vi "POST IoT Config Details.vi"(0 "GTron in":path, 3 "error in":errorcluster) -> (6 "IsEmpty":bool, 9 "error out":errorcluster)   [LabVIEW 2019, in "DataLogger.lvclass"]
doc: "POST IoT Configuration Details"
uses:
  DataLogger.lvclass
  <vilib>/drjdpowell/SQLite Library/SQL Connection/Execute SQL (Single Integer).vi
  <vilib>/httpClient/LabVIEWHTTPClient.lvlib
  <vilib>/drjdpowell/SQLite Library/SQL Statement/SQL Statement.lvclass
  <vilib>/drjdpowell/SQLite Library/SQL Connection/Execute SQL (No results).vi
  <vilib>/httpClient/POSTBuffer.vi
  <vilib>/drjdpowell/SQLite Library/SQL Connection/Open (path).vi
  <vilib>/drjdpowell/SQLite Library/SQL Connection/Connection.lvclass
panel:
  in  "IoT_Config Keys in":string[](array[string])=["ClientId", "ClientName", "Location", "NoOfShifts", "RunningShift", "ShiftTiming", "InspectionMcId", "IoTEnable", "SMSAlertEnable", "EmailAlertEnable", "PopUpEnable"]
  in  "Sever Info Cluster fot IoT Config":T1={"JSON Buffer"="authtoken=47244d7c61d7e6141acdddeabbf622d1&scope=creatorapi&zc_ownername=zentron3&XMLString=", "Server information start tag"="<ZohoCreator> <applicationlist> <application name='iiot-gtron'><formlist>  <form name='Iot_Config'>", "Record start/end"="add", "Key name"="field name", "Value name"="value", "Server information end tag"="\"</form></formlist></application></applicationlist></ZohoCreator>"}
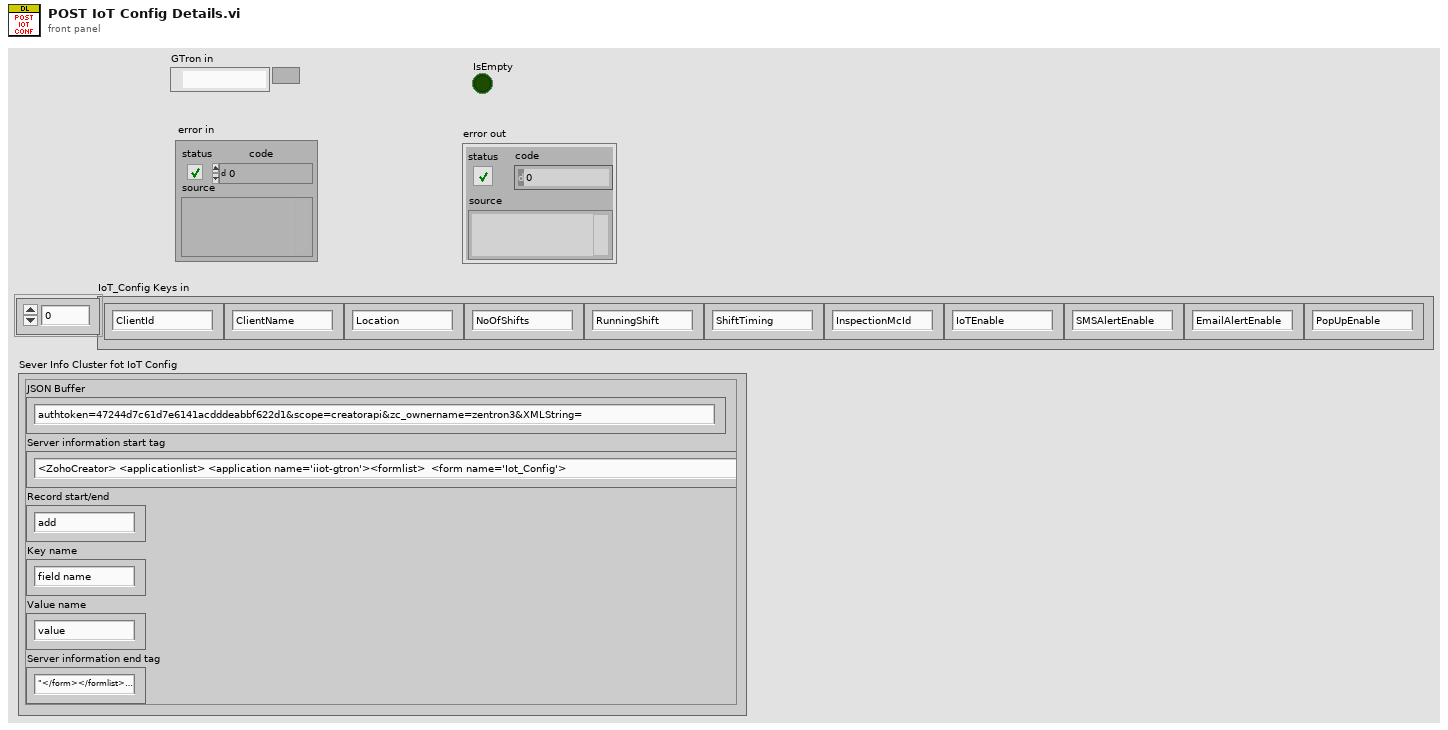
[diagram p1: front panel]
types:
  T1 = cluster{"JSON Buffer":string, "Server information start tag":string, "Record start/end":string, "Key name":string, "Value name":string, "Server information end tag":string}
  T2 = typedef "LabVIEWHTTPClient.lvlib/ClientHandle.ctl" = refnum<k1>
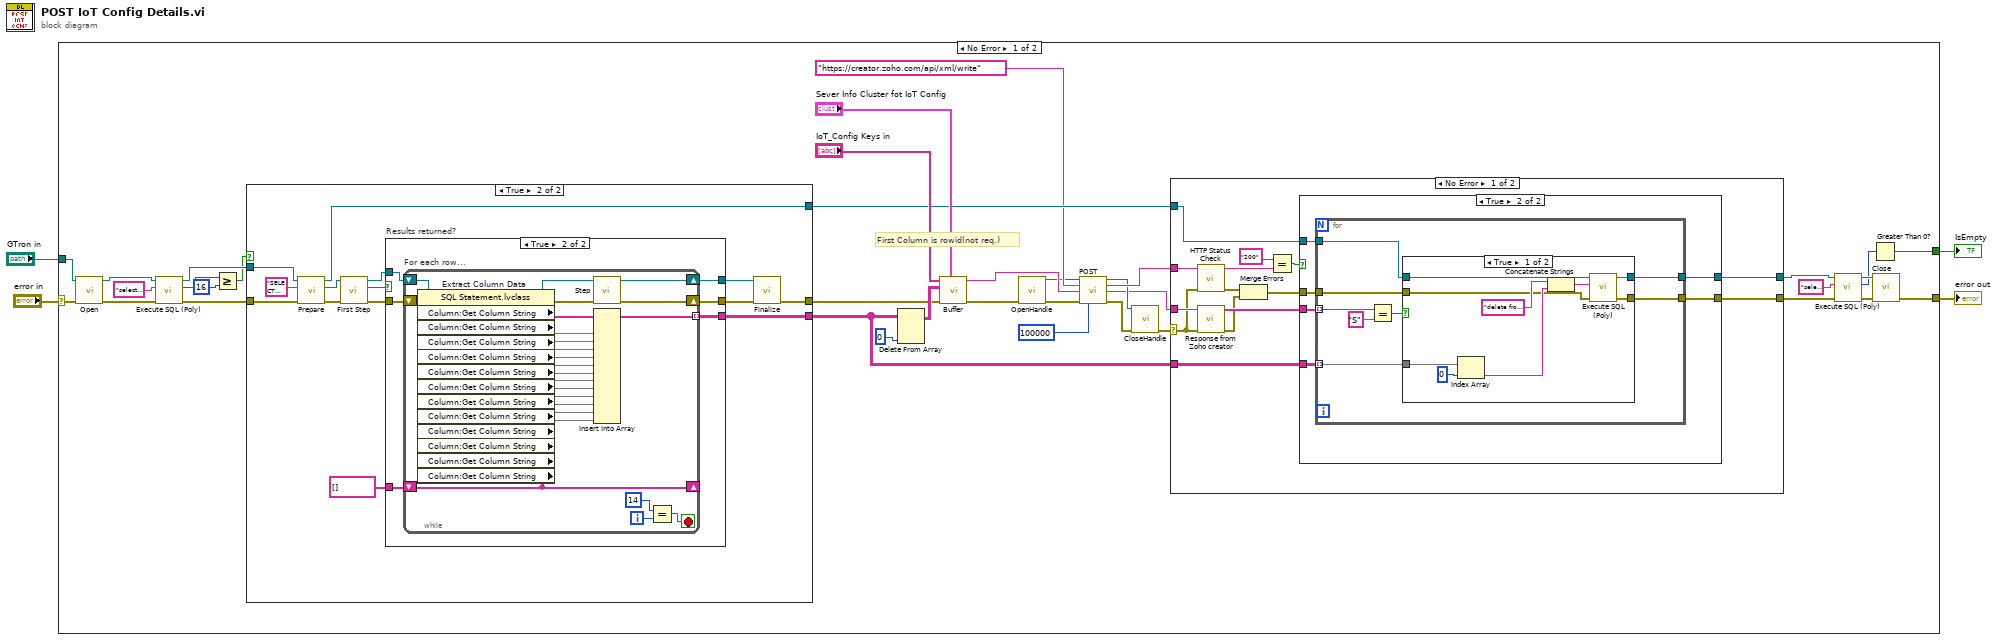
[diagram p0: block diagram]
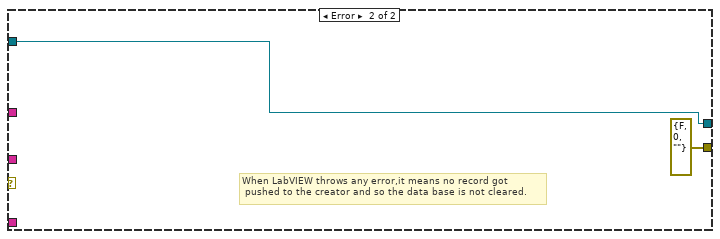
[diagram p4: hidden frame]
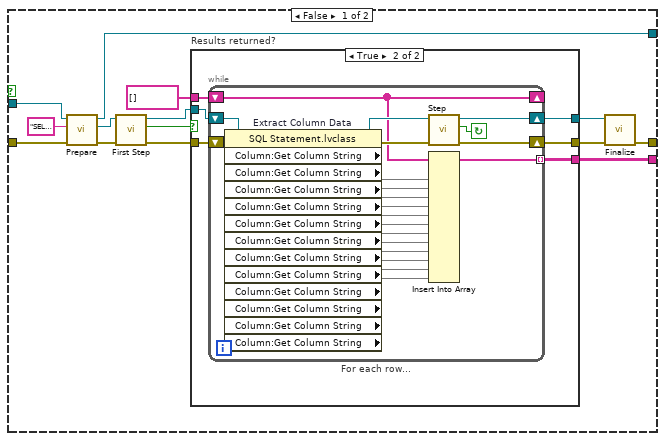
[diagram p5: hidden frame]
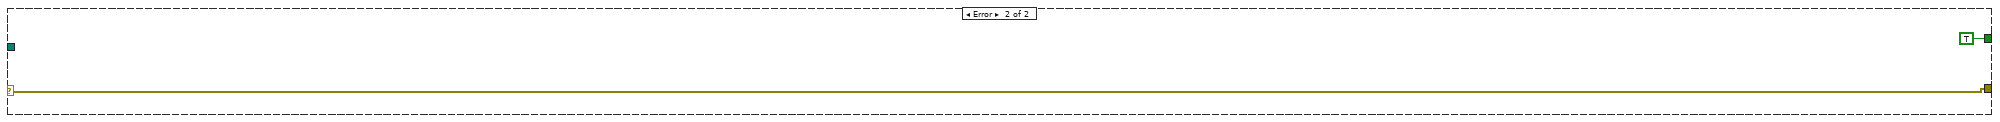
[diagram p8: hidden frame]
diagram:
  n1 = case shown="No Error" "error in" {
    selector: "error in" -> [w5 w172]
    tunnel: "GTron in" -> [w40 _]
    tunnel: [w39 w172] -> w3
    tunnel: [w6 TRUE] -> w2
    frame No Error {
      # "First Column is rowid(not req.)"
      n2 = call-poly <vilib>:"Open.vi"("error in (no error)"=w5, "db file"=w40) -> ("error out"=w37:errorcluster, "SQLite Connection"=w38:refnum<class "Connection.lvclass">)  [unwired: 8 in]
      n3 = call-poly <vilib>:"Execute SQL (Poly).vi"("error in (no error)"=w37, "SQL"="select count(*) from IoTConfigDetails ", "SQLite Connection in"=w38) -> ("error out"=w13:errorcluster, "Result"=w18:i64, "SQLite Connection"=w32:refnum<class "Connection.lvclass">)  [unwired: 6 in]
      n4 = Greater Or Equal?(x=w18, y=i64 16) -> (x >= y?=w20:bool)
      n5 = case shown="True" w20 {
        tunnel: [w89 w132] -> w34
        tunnel: w32 -> [w88 w131]
        tunnel: [w87 w130] -> w33
        tunnel: w13 -> [w85 w129]
        tunnel: [w86 w128] -> w16
        frame False {
          n6 = call <vilib>:"Prepare.vi"("error in (no error)"=w85, "SQL"="SELECT rowid,ClientId,ClientName,Location,NoOfShifts,RunningShift,ShiftTiming,InspectionMcId,IoTEnable,SMSAlertEnable,EmailAlertEnable,PopupEnable FROM IoTConfigDetails" ("SELECT  statement"), "SQLite Connection in"=w88) -> ("error out"=w96:errorcluster, "SQL Statement"=w92:refnum<class "SQL Statement.lvclass">, "SQLite Connection"=w87:refnum<class "Connection.lvclass">)  [unwired: 4 in, 2 out]
          n7 = call <vilib>:"First Step.vi"("error in (no error)"=w96, "SQL Statement in"=w92) -> ("error out"=w94:errorcluster, "Row returned"=w95:bool, "SQL Statement"=w93:refnum<class "SQL Statement.lvclass">)  [unwired: 7 in]
          n8 = case "Results returned?" shown="True" w95 {
            tunnel: [w99 w105] -> w91
            tunnel: [w98 w104] -> w90
            tunnel: w93 -> [w99 w103]
            tunnel: w94 -> [w98 w102]
            tunnel: string[] [] -> [_ w101]
            tunnel: [_ w100] -> w89
            frame False {
            }
            frame True {
              n9 = while "For each row..." {
                shift-right: [w125] -> w105
                shift-left: w103 -> [w122]
                shift-right: [w123] -> w104
                shift-left: w102 -> [w121]
                shift-right: [w107] -> _
                shift-left: w101 -> [w107]
                tunnel: [w113] -> w100 mode=indexing
                stop <- w111 continue-if-true
                n10 = property on="Extract Column Data" class="SQL Statement.lvclass"(reference=w122, error in=w121) -> (reference out=w126:refnum<class "SQL Statement.lvclass">, error out=w124:errorcluster, "Column:Get Column String"=w112, "Column:Get Column String"=w120, "Column:Get Column String"=w119, "Column:Get Column String"=w118, "Column:Get Column String"=w117, "Column:Get Column String"=w116, "Column:Get Column String"=w115, "Column:Get Column String"=w114, "Column:Get Column String"=w110, "Column:Get Column String"=w109, "Column:Get Column String"=w108, "Column:Get Column String"=w106)
                n11 = call <vilib>:"Step.vi"("error in (no error)"=w124, "SQL Statement in"=w126) -> ("error out"=w123:errorcluster, "Row returned"=w111:bool, "SQL Statement"=w125:refnum<class "SQL Statement.lvclass">)  [unwired: 7 in]
                n12 = Insert Into Array(array=w107, new element #1=w112, new element #2=w120, new element #3=w119, new element #4=w118, new element #5=w117, new element #6=w116, new element #7=w115, new element #8=w114, new element #9=w110, new element #10=w109, new element #11=w108, new element #12=w106) -> (w113:string[])  [unwired: 1 in]
              }
            }
          }
          n13 = call <vilib>:"Finalize.vi"("error in (no error)"=w90, "SQL Statement in"=w91) -> ("error out"=w86:errorcluster)  [unwired: 9 in]
        }
        frame True {
          n14 = call <vilib>:"Prepare.vi"("error in (no error)"=w129, "SQL"="SELECT rowid,ClientId,ClientName,Location,NoOfShifts,RunningShift,ShiftTiming,InspectionMcId,IoTEnable,SMSAlertEnable,EmailAlertEnable,PopupEnable FROM IoTConfigDetails" ("SELECT  statement"), "SQLite Connection in"=w131) -> ("error out"=w139:errorcluster, "SQL Statement"=w135:refnum<class "SQL Statement.lvclass">, "SQLite Connection"=w130:refnum<class "Connection.lvclass">)  [unwired: 4 in, 2 out]
          n15 = call <vilib>:"First Step.vi"("error in (no error)"=w139, "SQL Statement in"=w135) -> ("error out"=w137:errorcluster, "Row returned"=w138:bool, "SQL Statement"=w136:refnum<class "SQL Statement.lvclass">)  [unwired: 7 in]
          n16 = case "Results returned?" shown="True" w138 {
            tunnel: [w142 w148] -> w134
            tunnel: [w141 w147] -> w133
            tunnel: w136 -> [w142 w146]
            tunnel: w137 -> [w141 w145]
            tunnel: string[] [] -> [_ w144]
            tunnel: [_ w143] -> w132
            frame False {
            }
            frame True {
              n17 = while "For each row..." {
                shift-right: [w170] -> w148
                shift-left: w146 -> [w167]
                shift-right: [w168] -> w147
                shift-left: w145 -> [w166]
                shift-right: [w165] -> _
                shift-left: w144 -> [w165]
                tunnel: [w157] -> w143 mode=indexing
                i -> [w156]
                stop <- w154 stop-if-true
                n18 = property on="Extract Column Data" class="SQL Statement.lvclass"(reference=w167, error in=w166) -> (reference out=w171:refnum<class "SQL Statement.lvclass">, error out=w169:errorcluster, "Column:Get Column String"=w153, "Column:Get Column String"=w164, "Column:Get Column String"=w163, "Column:Get Column String"=w162, "Column:Get Column String"=w161, "Column:Get Column String"=w160, "Column:Get Column String"=w159, "Column:Get Column String"=w158, "Column:Get Column String"=w152, "Column:Get Column String"=w151, "Column:Get Column String"=w150, "Column:Get Column String"=w149)
                n19 = call <vilib>:"Step.vi"("error in (no error)"=w169, "SQL Statement in"=w171) -> ("error out"=w168:errorcluster, "SQL Statement"=w170:refnum<class "SQL Statement.lvclass">)  [unwired: 7 in, 1 out]
                n20 = Insert Into Array(array=w165, new element #1=w153, new element #2=w164, new element #3=w163, new element #4=w162, new element #5=w161, new element #6=w160, new element #7=w159, new element #8=w158, new element #9=w152, new element #10=w151, new element #11=w150, new element #12=w149) -> (w157:string[])  [unwired: 1 in]
                n21 = Equal?(x=14, y=w156) -> (x = y?=w154:bool)
              }
            }
          }
          n22 = call <vilib>:"Finalize.vi"("error in (no error)"=w133, "SQL Statement in"=w134) -> ("error out"=w128:errorcluster)  [unwired: 9 in]
        }
      }
      n23 = Delete From Array(array=w34, index (col)=0 ("disabled index (col)")) -> (array with subset deleted=w22:string[][])  [unwired: 2 in, 1 out]
      n24 = call "Buffer.vi"("Cluster"="Sever Info Cluster fot IoT Config", "error in"=w16, "Values"=w22, "Keys"="IoT_Config Keys in") -> ("Error out"=w15:errorcluster, "Buffer"=w25:string)  [unwired: 6 in]
      n25 = call <vilib>:"OpenHandle.vi"("error in (no error)"=w15) -> ("client handle out"=w23:T2, "error out"=w28:errorcluster)  [unwired: 13 in]
      n26 = call-poly <vilib>:"POST.vi"("client handle"=w23, "url"="https://creator.zoho.com/api/xml/write", "buffer"=w25, "error in (no error)"=w28, "timeout (10000)"=100000) -> ("client handle out"=w24:T2, "headers"=w31:string, "body"=w14:string, "error out"=w29:errorcluster)  [unwired: 7 in]
      n27 = call <vilib>:"CloseHandle.vi"("client handle"=w24, "error in (no error)"=w29) -> ("error out"=w30:errorcluster)  [unwired: 13 in]
      n28 = case shown="No Error" w30 {
        selector: w30 -> [w44 _]
        tunnel: w31 -> [w54 _]
        tunnel: w33 -> [w50 w83]
        tunnel: w34 -> [w49 _]
        tunnel: [w48 w83] -> w10
        tunnel: [w47 errorcluster {"status"=FALSE, "code"=0, "source"=""} ("error out")] -> w11
        tunnel: w14 -> [w45 _]
        frame No Error {
          n29 = call "HTTP Status Check.vi"("error in (no error)"=w44, "String"=w54) -> ("error out"=w42:errorcluster, "HTTP Status Code"=w53:string)  [unwired: 7 in]
          n30 = call "Response from Zoho creator.vi"("error in"=w44, "body"=w45) -> ("error out"=w41:errorcluster, "decimated array"=w46:string[])  [unwired: 8 in]
          n31 = Merge Errors(w42, w41) -> (w43:errorcluster)
          n32 = Equal?(x="200" ("y"), y=w53) -> (x = y?=w51:bool)
          n33 = case shown="True" w51 {
            tunnel: w46 -> [_ w61]
            tunnel: w50 -> [w56 w62]
            tunnel: w49 -> [_ w60]
            tunnel: [w56 w59] -> w48
            tunnel: w43 -> [w55 w58]
            tunnel: [w55 w57] -> w47
            frame False {
              # "When HTTP Status is anything except 200,it means no record\ngot pushed to the creator and so the database is not cleared"
            }
            frame True {
              n34 = for {
                tunnel: w62 -> [w70]
                tunnel: w60 -> [w66] mode=indexing
                tunnel: w61 -> [w69] mode=indexing
                tunnel: [w65] -> w59
                tunnel: w58 -> [w64]
                tunnel: [w63] -> w57
                n35 = Equal?(x=w69, y="S") -> (x = y?=w67:bool)
                n36 = case shown="True" w67 {
                  tunnel: w70 -> [w79 w81]
                  tunnel: w66 -> [w78 _]
                  tunnel: [w73 w81] -> w65
                  tunnel: w64 -> [w72 w80]
                  tunnel: [w71 w80] -> w63
                  frame True {
                    n37 = Index Array(array=w78, index=0) -> (element=w76:string)
                    n38 = Concatenate Strings("delete from IoTConfigDetails where rowid = " ("SQL"), w76) -> (w74:string)
                    n39 = call-poly <vilib>:"Execute SQL (Poly).vi"("error in (no error)"=w72, "SQL"=w74, "SQLite Connection in"=w79) -> ("error out"=w71:errorcluster, "SQLite Connection"=w73:refnum<class "Connection.lvclass">)  [unwired: 7 in]
                  }
                  frame False {
                  }
                }
              }
            }
          }
        }
        frame Error {
          # "When LabVIEW throws any error,it means no record got\n pushed to the creator and so the data base is not cleared."
        }
      }
      n40 = call-poly <vilib>:"Execute SQL (Poly).vi"("error in (no error)"=w11, "SQL"="select count(*) from IoTConfigDetails ", "SQLite Connection in"=w10) -> ("error out"=w12:errorcluster, "Result"=w7:i64, "SQLite Connection"=w9:refnum<class "Connection.lvclass">)  [unwired: 6 in]
      n41 = Greater Than 0?(x=w7) -> (x > 0?=w6:bool)
      n42 = call-dynamic "Close.vi"("error in (no error)"=w12, "SQLite Connection in"=w9) -> ("error out"=w39:errorcluster)  [unwired: 9 in]
    }
    frame Error {
    }
  }
  "error out" <- w3
  "IsEmpty" <- w2
